vi "Calc Channel Format.vi"(8 "error in":errorcluster, 9 "Format":i32(ring) items=["Linear", "Log", "Phase", "Real", "Imaginary"], 10 "Calc Channel":i32(ring) caption="Calculation Channel" items=["Calc Channel 1", "Calc Channel 2", "Calc Channel 3", "Calc Channel 4"], 11 "Instrument Handle In":i32) -> (0 "error out":errorcluster, 3 "Instrument Handle Out":i32)   [LabVIEW 8.6, in "ZTScopeM.lvlib"]
doc: "Configure the data format of the selected calculation channel. This only applies to frequency based waveforms (FFTs)."
uses:
  ZTScopeM.lvlib
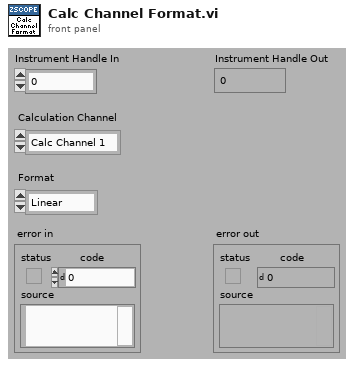
[diagram p1: front panel]
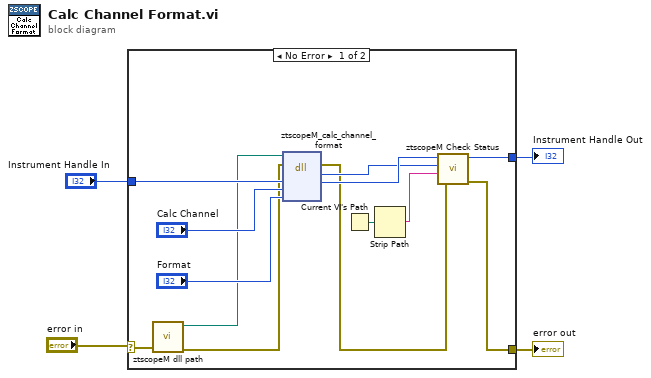
[diagram p0: block diagram]
diagram:
  n1 = case shown="No Error" "error in" {
    selector: "error in" -> [w8 w19]
    tunnel: [w10 w19] -> w1
    tunnel: "Instrument Handle In" -> [w17 w18]
    tunnel: [w9 w18] -> w3
    frame #0 {
      n2 = call "ztscopeM dll path.vi"("error in (no error)"=w8) -> ("error out"=w6:errorcluster, "<instrument>.dll path"=w7:path)  [unwired: 9 in]
      n3 = dll-call lib="C:/Program Files (x86)/National Instruments/LabVIEW 2013/instr.lib/ztscopem/ztscopeM.dll" fn="ztscopeM_calc_channel_format"(path in=w7, error in=w6, "instrumentHandle"=w17, "calculationChannel"="Calc Channel", "format"="Format") -> (error out=w5:errorcluster, w11:i32, "instrumentHandle"=w12:i32)  [unwired: 3 in, 1 out]
      n4 = Current VI's Path() -> (path=w14:path)
      n5 = Strip Path(path=w14) -> (name=w13:string)  [unwired: 1 out]
      n6 = call "ztscopeM Check Status.vi"("error in"=w5, "name of VI"=w13, "status (return code)"=w11, "instrument handle in"=w12) -> ("error out"=w10:errorcluster, "instrument handle out"=w9:i32)  [unwired: 2 in]
    }
    frame #1 {
    }
  }
  "Instrument Handle Out" <- w3
  "error out" <- w1
